vi "HoloPy_set_hologram.vi"(8 "error in (no error)":errorcluster, 9 "HOLO_array":sgl[][](array[numeric]), 11 "Refnum in":refnum<k35>) -> (0 "error out":errorcluster, 1 "return value":string, 3 "Refnum out":refnum<k35>)   [LabVIEW 2025, in "holoTracker.lvlib"]
uses:
  holoTracker.lvlib
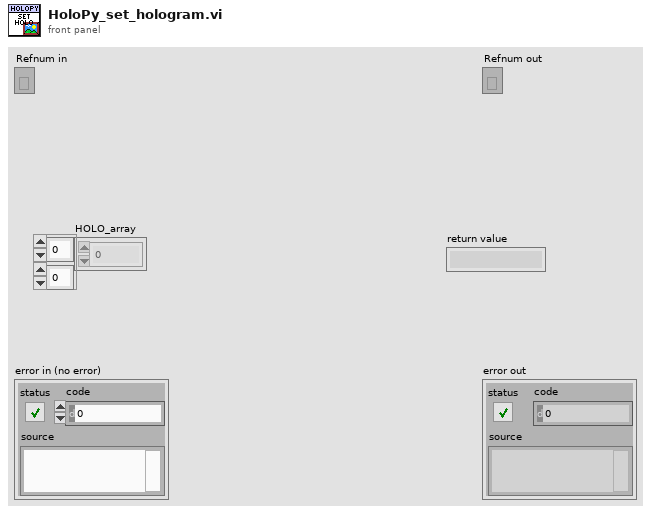
[diagram p1: front panel]
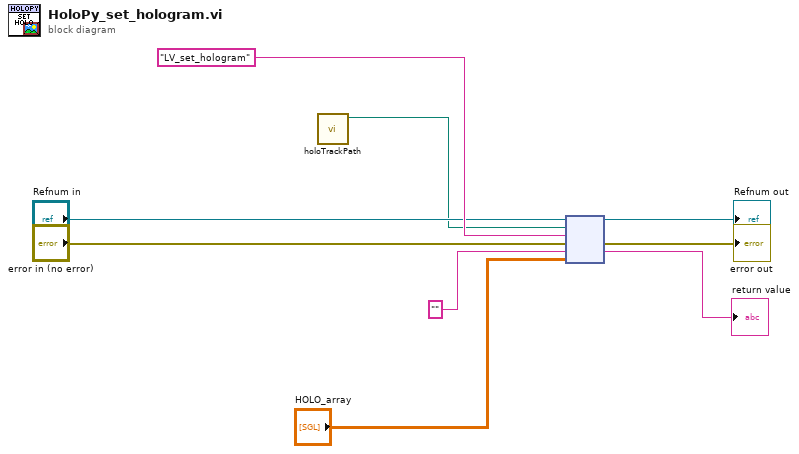
[diagram p0: block diagram]
diagram:
  n1 = call "holoTrackPath.vi"() -> ("appended path"=w1:path)  [unwired: 11 in]
  n2 = node("Refnum in", w1, "LV_set_hologram" ("function name"), "error in (no error)", "", "HOLO_array") -> (→"Refnum out":refnum<k35>, →"error out":errorcluster, →"return value":string)  [unwired: 1 in, 2 out]
